vi "Facade Line Chart.vi"(0 "Data In":T4, 2 "Display State In":T2, 3 "Container State":T3) -> (6 "Data Out":T4, 7 "Display State Out":T2, 8 "Action":T1)   [LabVIEW 2016, in "Line Chart.xctl"]
uses:
  Line Chart.xctl
  Data Line Chart.ctl
  <vilib>/_xctls/Container State.ctl
  State Line Chart.ctl
  <vilib>/_xctls/Action.ctl
  <vilib>/_xctls/XControlSupport.lvlib
panel:
  in  "ActiveX Container":refnum<k7>(container)
types:
  T1 = typedef "XControlSupport.lvlib/Action.ctl" = cluster{"Data Changed?":bool, "State Changed?":bool, "Action Name":string}
  T2 = typedef "Line Chart.xctl/State Line Chart.ctl" = cluster{"Numeric":dbl}
  T3 = typedef "XControlSupport.lvlib/Container State.ctl" = cluster{"Indicator?":bool, "Run Mode?":bool, " Refnum":refnum<vi>}
  T4 = typedef "Line Chart.xctl/Data Line Chart.ctl" = cluster{"X-Axis":string[], "Plots":cluster{"Data":dbl[], "Label":string, "Y-Axis":enum16{"Y-Axis 1", "Y-Axis 2", "Y-Axis 3", "Y-Axis 4", "Y-Axis 5", "Y-Axis 6", "Y-Axis 7", "Y-Axis 8", "Y-Axis 9", "Y-Axis 10"}, "Color":u32, "unit":string}[], "Plot Title":string}
  T5 = enum32{"invalid app kind", "Development System", "Run Time System", "Student Edition", "Embedded LabVIEW", "Evaluation", "Custom"}
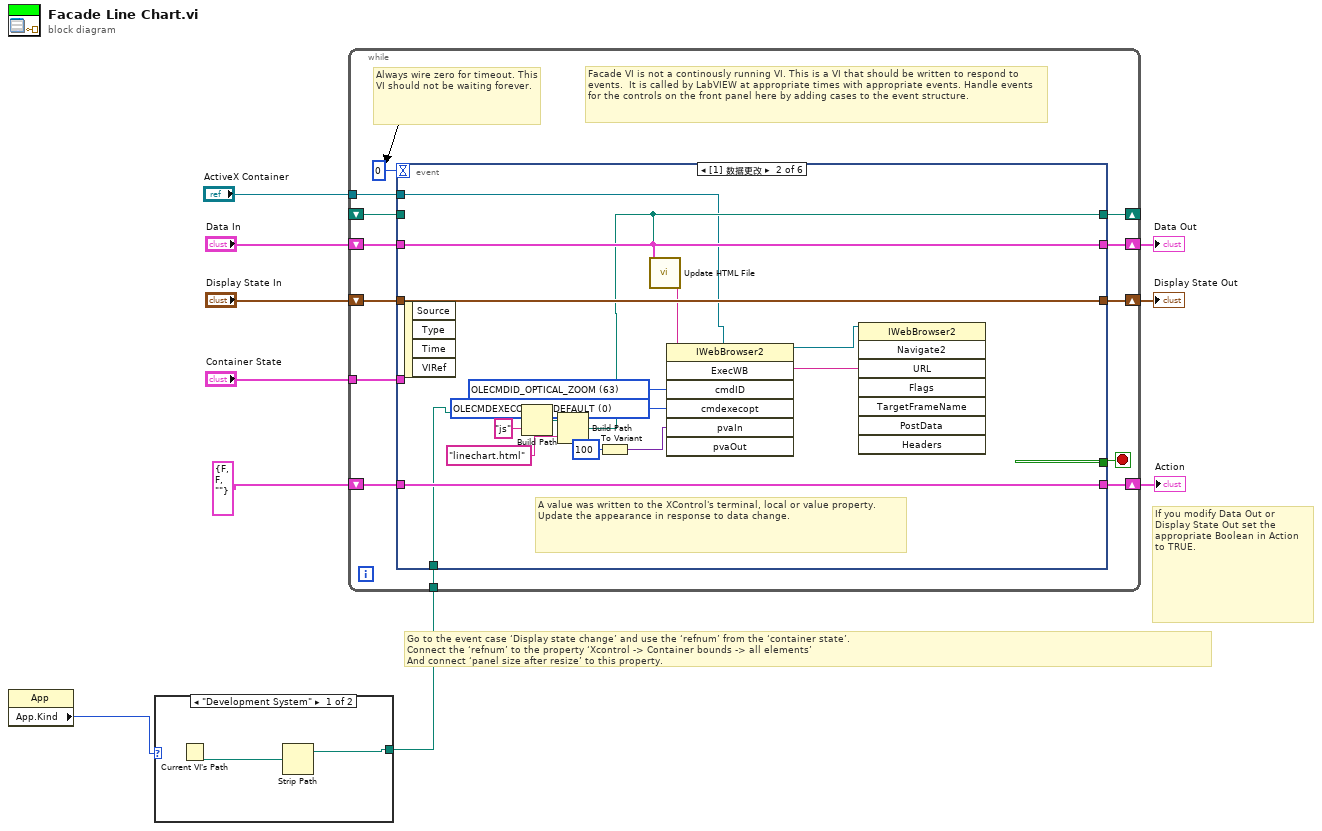
[diagram p0: block diagram]
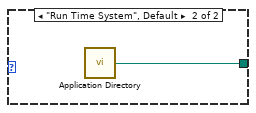
[diagram p2: hidden frame]
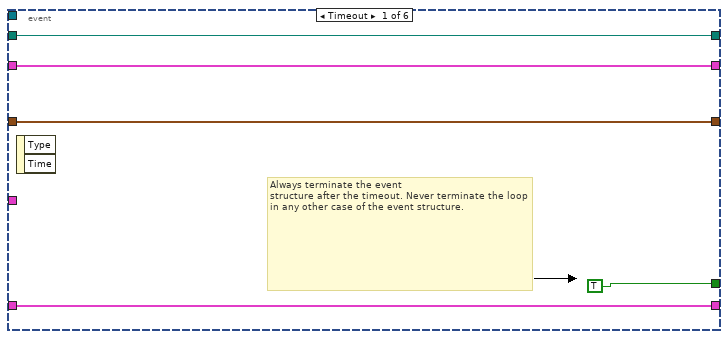
[diagram p3: hidden frame]
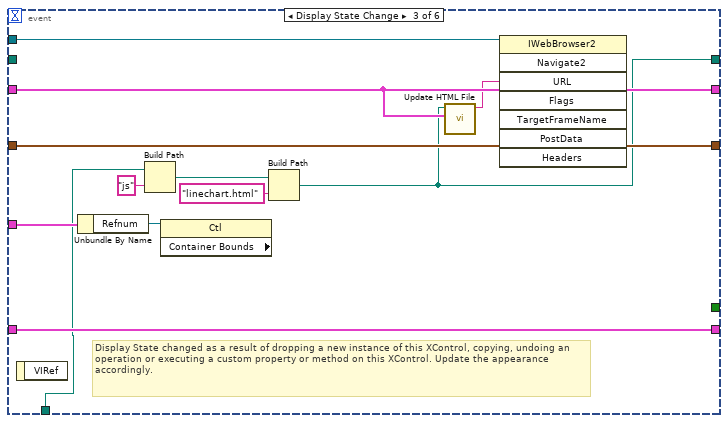
[diagram p4: hidden frame]
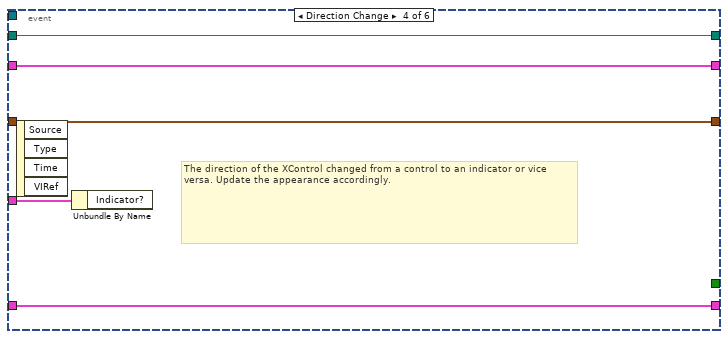
[diagram p5: hidden frame]
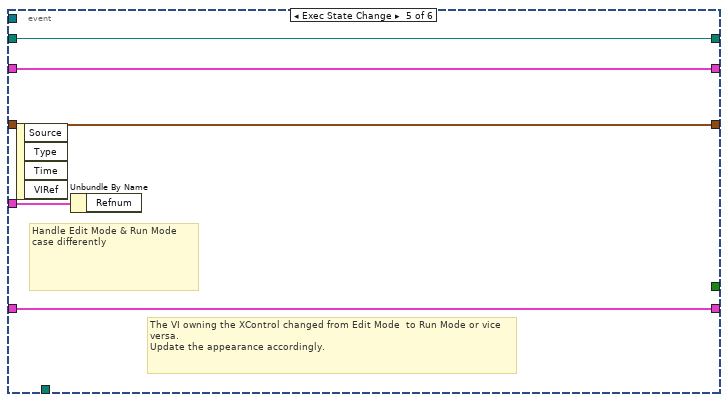
[diagram p6: hidden frame]
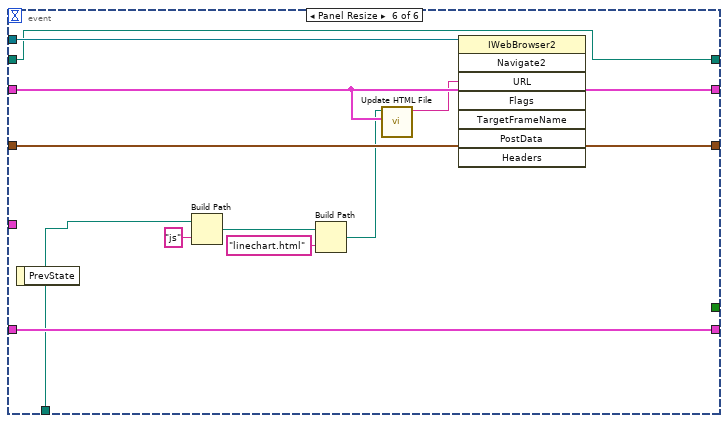
[diagram p7: hidden frame]
diagram:
  # "Go to the event case ‘Display state change’ and use the ‘refnum’ from the ‘container state’.\nConnect the ‘refnum’ to the property ‘Xcontrol -> Container bounds -> all elements’\nAnd connect ‘panel size after resize’ to this property."
  # "If you modify Data Out or\nDisplay State Out set the\nappropriate Boolean in Action\nto TRUE."
  n1 = property class="App"() -> ("App.Kind"=w2:T5)  [unwired: 2 in, 2 out]
  n2 = case shown="\"Development System\"" w2 {
    tunnel: [w11 w13] -> w1
    frame "Development System" {
      n3 = Current VI's Path() -> (path=w12:path)
      n4 = Strip Path(path=w12) -> (stripped path=w11:path)  [unwired: 1 out]
    }
    frame "Run Time System", Default {
      n5 = call <vilib>:"Application Directory.vi"() -> ("Application Directory"=w13:path)
    }
  }
  n6 = while {
    shift-right: [w25] -> w7
    shift-left: "Display State In" -> [w26]
    tunnel: "Container State" -> [w22]
    shift-right: [w20] -> w10
    shift-left: "Data In" -> [w21]
    shift-right: [w18] -> w5
    shift-left: T1 {"Data Changed?"=FALSE, "State Changed?"=FALSE, "Action Name"=""} ("Action") -> [w19]
    tunnel: "ActiveX Container" -> [w17]
    shift-right: [w16] -> _
    shift-left: _ -> [w15]
    tunnel: w1 -> [w14]
    stop <- w24 stop-if-true
    # "Facade VI is not a continously running VI. This is a VI that should be written to respond to events.  It is called by LabVIEW at appropriate times with appropriate events. Handle events for the controls on the front panel here by adding cases to the event structure."
    # "Always wire zero for timeout. This\nVI should not be waiting forever."
    n7 = event shown="[1] 数据更改" {
      selector: _ -> [_ _ _ _ _ _]
      dyn-events: _ -> [_ _ _ _ _ _]
      timeout: 0 -> [_ _ _ _ _ _]
      tunnel: w26 -> [w29 w46 w58 w62 w67 w79]
      tunnel: [w29 w46 w58 w62 w67 w79] -> w25
      tunnel: [TRUE _ _ _ _ _] -> w24
      tunnel: w22 -> [_ _ w56 w63 w68 _]
      tunnel: w21 -> [w28 w44 w51 w61 w66 w76]
      tunnel: [w28 w44 w51 w61 w66 w76] -> w20
      tunnel: [w30 w45 w57 w60 w65 w78] -> w18
      tunnel: w19 -> [w30 w45 w57 w60 w65 w78]
      tunnel: w17 -> [_ w37 w47 _ _ w77]
      tunnel: [w27 w43 w50 w59 w64 w75] -> w16
      tunnel: w15 -> [w27 _ _ w59 w64 w75]
      tunnel: w14 -> [_ w38 w48 _ _ w69]
      event Timeout {
        # "Always terminate the event\nstructure after the timeout. Never terminate the loop in any other case of the event structure."
        n8 = event-data() -> ()  [unwired: 1 in, 2 out]
      }
      event Data Change {
        w32 = 0 items=["OLECMDEXECOPT_DODEFAULT", "OLECMDEXECOPT_PROMPTUSER", "OLECMDEXECOPT_DONTPROMPTUSER", "OLECMDEXECOPT_SHOWHELP"] ("cmdexecopt")
        w35 = 63 items=["OLECMDID_OPEN"=1, "OLECMDID_NEW"=2, "OLECMDID_SAVE"=3, "OLECMDID_SAVEAS"=4, "OLECMDID_SAVECOPYAS"=5, "OLECMDID_PRINT"=6, "OLECMDID_PRINTPREVIEW"=7, "OLECMDID_PAGESETUP"=8, "OLECMDID_SPELL"=9, "OLECMDID_PROPERTIES"=10, "OLECMDID_CUT"=11, "OLECMDID_COPY"=12, "OLECMDID_PASTE"=13, "OLECMDID_PASTESPECIAL"=14, "OLECMDID_UNDO"=15, "OLECMDID_REDO"=16, "OLECMDID_SELECTALL"=17, "OLECMDID_CLEARSELECTION"=18, "OLECMDID_ZOOM"=19, "OLECMDID_GETZOOMRANGE"=20, "OLECMDID_UPDATECOMMANDS"=21, "OLECMDID_REFRESH"=22, "OLECMDID_STOP"=23, "OLECMDID_HIDETOOLBARS"=24, "OLECMDID_SETPROGRESSMAX"=25, "OLECMDID_SETPROGRESSPOS"=26, "OLECMDID_SETPROGRESSTEXT"=27, "OLECMDID_SETTITLE"=28, "OLECMDID_SETDOWNLOADSTATE"=29, "OLECMDID_STOPDOWNLOAD"=30, "OLECMDID_ONTOOLBARACTIVATED"=31, "OLECMDID_FIND"=32, "OLECMDID_DELETE"=33, "OLECMDID_HTTPEQUIV"=34, "OLECMDID_HTTPEQUIV_DONE"=35, "OLECMDID_ENABLE_INTERACTION"=36, "OLECMDID_ONUNLOAD"=37, "OLECMDID_PROPERTYBAG2"=38, "OLECMDID_PREREFRESH"=39, "OLECMDID_SHOWSCRIPTERROR"=40, "OLECMDID_SHOWMESSAGE"=41, "OLECMDID_SHOWFIND"=42, "OLECMDID_SHOWPAGESETUP"=43, "OLECMDID_SHOWPRINT"=44, "OLECMDID_CLOSE"=45, "OLECMDID_ALLOWUILESSSAVEAS"=46, "OLECMDID_DONTDOWNLOADCSS"=47, "OLECMDID_UPDATEPAGESTATUS"=48, "OLECMDID_PRINT2"=49, "OLECMDID_PRINTPREVIEW2"=50, "OLECMDID_SETPRINTTEMPLATE"=51, "OLECMDID_GETPRINTTEMPLATE"=52, "OLECMDID_PAGEACTIONBLOCKED"=55, "OLECMDID_PAGEACTIONUIQUERY"=56, "OLECMDID_FOCUSVIEWCONTROLS"=57, "OLECMDID_FOCUSVIEWCONTROLSQUERY"=58, "OLECMDID_SHOWPAGEACTIONMENU"=59, "OLECMDID_ADDTRAVELENTRY"=60, "OLECMDID_UPDATETRAVELENTRY"=61, "OLECMDID_UPDATEBACKFORWARDSTATE"=62, "OLECMDID_OPTICAL_ZOOM"=63, "OLECMDID_OPTICAL_GETZOOMRANGE"=64, "OLECMDID_WINDOWSTATECHANGED"=65, "OLECMDID_ACTIVEXINSTALLSCOPE"=66, "OLECMDID_UPDATETRAVELENTRY_DATARECOVERY"=67, "OLECMDID_SHOWTASKDLG"=68, "OLECMDID_POPSTATEEVENT"=69, "OLECMDID_VIEWPORT_MODE"=70, "OLECMDID_LAYOUT_VIEWPORT_WIDTH"=71, "OLECMDID_VISUAL_VIEWPORT_EXCLUDE_BOTTOM"=72, "OLECMDID_USER_OPTICAL_ZOOM"=73, "OLECMDID_PAGEAVAILABLE"=74, "OLECMDID_GETUSERSCALABLE"=75, "OLECMDID_UPDATE_CARET"=76, "OLECMDID_ENABLE_VISIBILITY"=77, "OLECMDID_MEDIA_PLAYBACK"=78, "OLECMDID_SETFAVICON"=79, "OLECMDID_SET_HOST_FULLSCREENMODE"=80, "OLECMDID_EXITFULLSCREEN"=81, "OLECMDID_SCROLLCOMPLETE"=82, "OLECMDID_ONBEFOREUNLOAD"=83, "OLECMDID_SHOWMESSAGE_BLOCKABLE"=84, "OLECMDID_SHOWTASKDLG_BLOCKABLE"=85] ("cmdID")
        # "A value was written to the XControl's terminal, local or value property.\nUpdate the appearance in response to data change."
        n9 = event-data() -> ()  [unwired: 1 in, 4 out]
        n10 = Build Path(base path=w38, name or relative path="js") -> (appended path=w41:path)
        n11 = Build Path(base path=w41, name or relative path="linechart.html") -> (appended path=w43:path)
        n12 = To Variant(anything=100) -> (Variant=w34:variant)
        n13 = call "Update HTML File.vi"("Data In"=w44, "Path"=w43) -> ("URL out"=w39:string)  [unwired: 9 in]
        n14 = invoke class="IWebBrowser2" method="ExecWB"(reference=w37, "cmdID"=w35, "cmdexecopt"=w32, "pvaIn"=w34) -> (reference out=w36:refnum<k7>)  [unwired: 3 in, 6 out]
        n15 = invoke class="IWebBrowser2" method="Navigate2"(reference=w36, "URL"=w39) -> ()  [unwired: 6 in, 8 out]
      }
      event Display State Change {
        # "Display State changed as a result of dropping a new instance of this XControl, copying, undoing an operation or executing a custom property or method on this XControl. Update the appearance accordingly."
        n16 = event-data() -> ()  [unwired: 1 in, 1 out]
        n17 = Unbundle By Name(w56) -> ("Refnum"=w52:refnum<vi>)
        n18 = Build Path(base path=w48, name or relative path="js") -> (appended path=w54:path)
        n19 = property class="Ctl" props=["Container Bounds"](reference=w52) -> ()  [unwired: 1 in, 3 out]
        n20 = Build Path(base path=w54, name or relative path="linechart.html") -> (appended path=w50:path)
        n21 = call "Update HTML File.vi"("Data In"=w51, "Path"=w50) -> ("URL out"=w49:string)  [unwired: 9 in]
        n22 = invoke class="IWebBrowser2" method="Navigate2"(reference=w47, "URL"=w49) -> ()  [unwired: 6 in, 8 out]
      }
      event Direction Change {
        # "The direction of the XControl changed from a control to an indicator or vice versa. Update the appearance accordingly."
        n23 = event-data() -> ()  [unwired: 1 in, 4 out]
        n24 = Unbundle By Name(w63) -> ()  [unwired: 1 out]
      }
      event Exec State Change {
        # "The VI owning the XControl changed from Edit Mode  to Run Mode or vice versa.\nUpdate the appearance accordingly."
        # "Handle Edit Mode & Run Mode\ncase differently"
        n25 = event-data() -> ()  [unwired: 1 in, 4 out]
        n26 = Unbundle By Name(w68) -> ()  [unwired: 1 out]
      }
      event Panel Resize {
        n27 = event-data() -> ()  [unwired: 1 in, 1 out]
        n28 = Build Path(base path=w69, name or relative path="js") -> (appended path=w72:path)
        n29 = Build Path(base path=w72, name or relative path="linechart.html") -> (appended path=w70:path)
        n30 = call "Update HTML File.vi"("Data In"=w76, "Path"=w70) -> ("URL out"=w74:string)  [unwired: 9 in]
        n31 = invoke class="IWebBrowser2" method="Navigate2"(reference=w77, "URL"=w74) -> ()  [unwired: 6 in, 8 out]
      }
    }
  }
  "Display State Out" <- w7
  "Data Out" <- w10
  "Action" <- w5
